vi "测试-掉线统计.vi"() -> ()   [LabVIEW 2017]
uses:
  <vilib>/Utility/miscctls.llb/LVRowAndColumnUnsignedTypeDef.ctl
panel:
  in  "标志-主动高亮":bool=TRUE
  in  "标志-刷新设备":bool=TRUE
  in  "清空记录":bool
  out "信号-高亮选中":bool=TRUE
  out "事件-新掉线记录":refnum<user-event>
  in  "掉线缓存":T1[](array[typedef])
  out "掉线记录":i32[](listbox)
  in  "设备":i32(listbox)
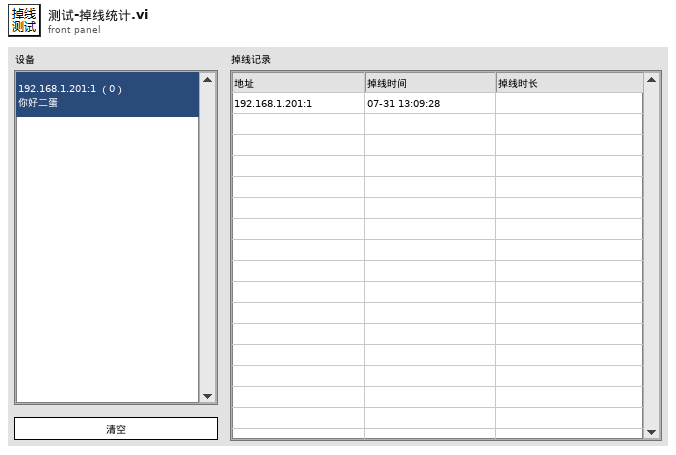
[diagram p1: front panel]
types:
  T1 = typedef "掉线缓存.ctl" = cluster{"掉线时长":string, "探头信息":cluster{"网络地址":string, "名称":string}, "掉线时间":timestamp, "记次":u16}
  T2 = typedef "LVRowAndColumnUnsignedTypeDef.ctl" = cluster{"Row":u32, "Column":u32}
  T3 = enum32{"Invalid", "Standard", "Closed", "Hidden", "Minimized", "Maximized"}
  T4 = typedef "探头属性.ctl" = cluster{"探头地址与信息":T5, "测量值":T8, "限值":T9, "探头状态":T10, "累积记录":T11, "报警方式":T12}
  T5 = typedef "探测器信息.ctl" = cluster{"网络地址":string, "名称":string, "备注":string, "累积剂量":dbl, "累积限值":dbl, "硬件剂量率限值":T6, "剂量率限值1":dbl, "剂量率限值2":dbl, "报警方式":T7}
  T6 = typedef "探头剂量率限值选择.ctl" = enum16{"一级限值", "二级限值"}
  T7 = typedef "报警方式选择.ctl" = enum16{"常报警", "自动静音", "手动静音"}
  T8 = typedef "测量值.ctl" = cluster{"时间":timestamp, "数值":dbl}
  T9 = typedef "剂量率限值.ctl" = cluster{"限值1":dbl, "限值2":dbl, "探头限值":T6}
  T10 = typedef "探头状态.ctl" = enum16{"正常", "离线", "禁用", "一级报警", "二级报警", "累积报警"}
  T11 = typedef "单条累积记录.ctl" = cluster{"起始时间":timestamp, "结束时间":timestamp, "累积剂量":dbl}
  T12 = typedef "报警方式.ctl" = cluster{"报警方式":T7, "延迟计时":u16, "报警中？":bool}
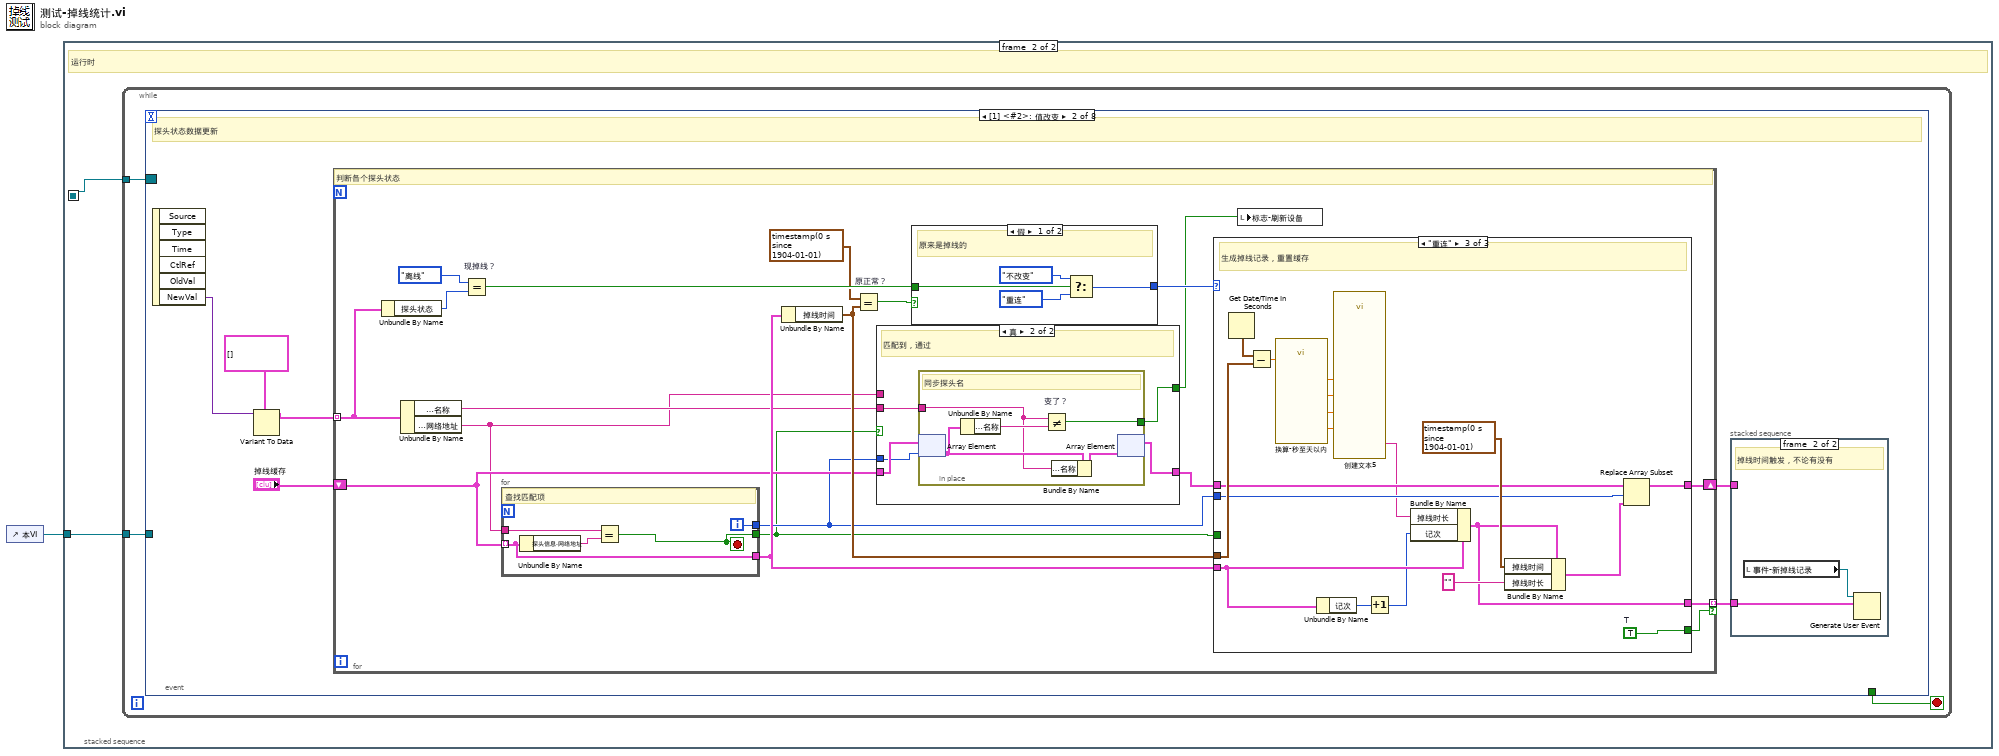
[diagram p0: block diagram]
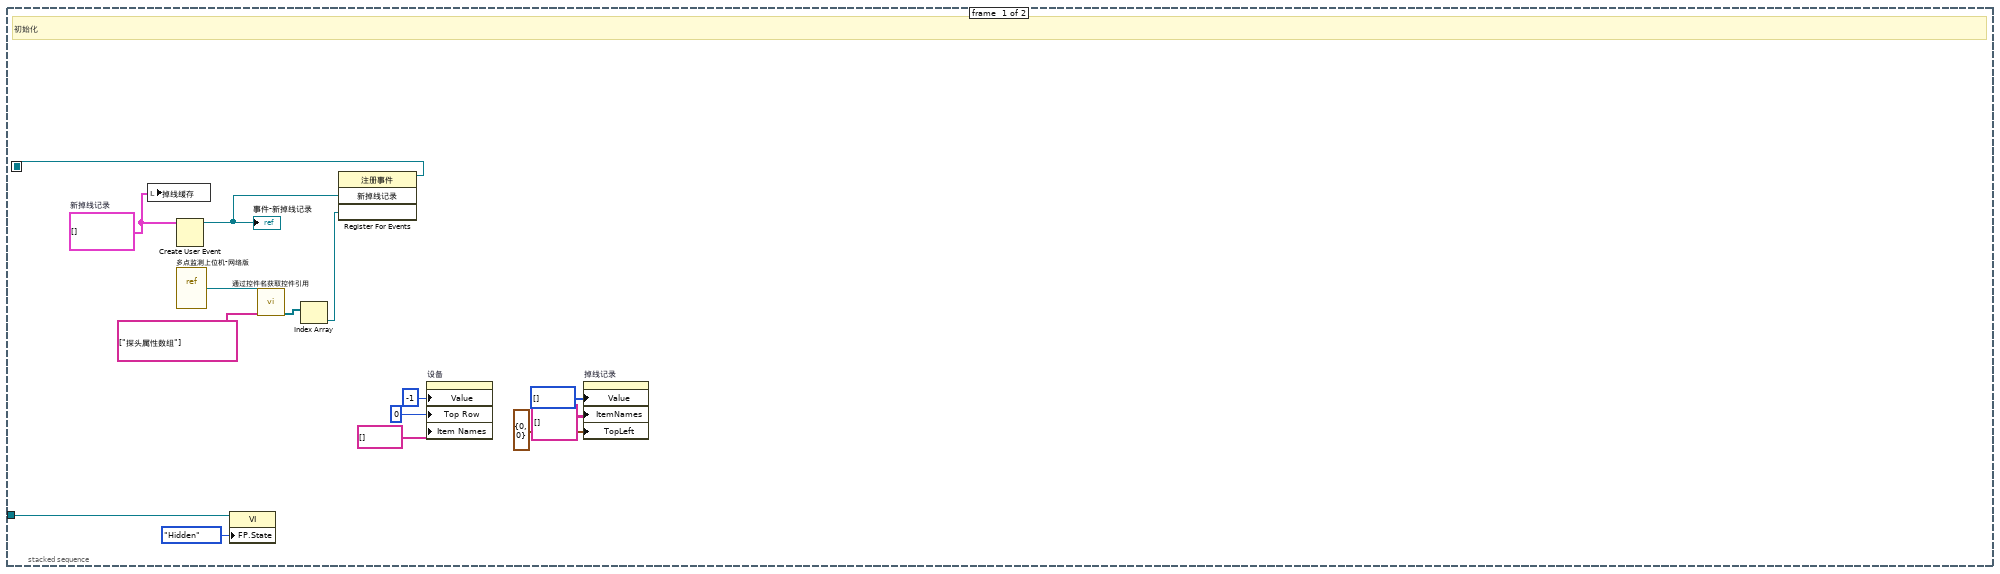
[diagram p2: hidden frame]
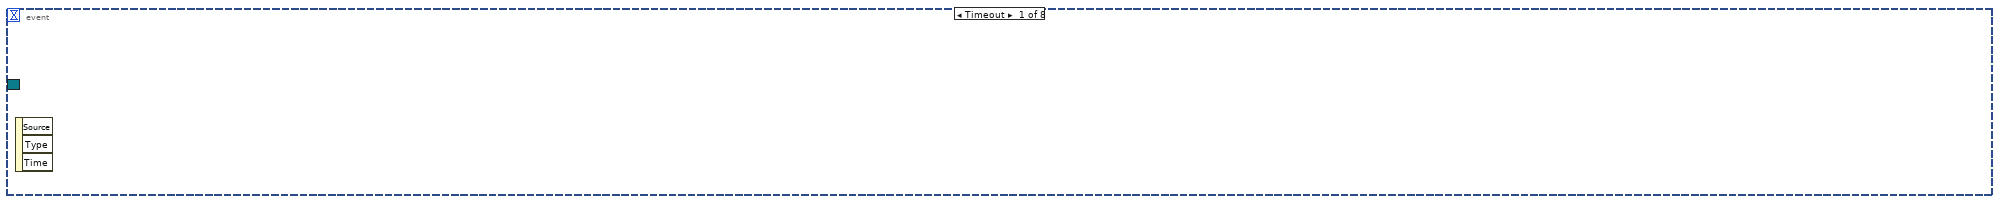
[diagram p3: hidden frame]
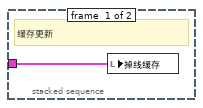
[diagram p4: hidden frame]
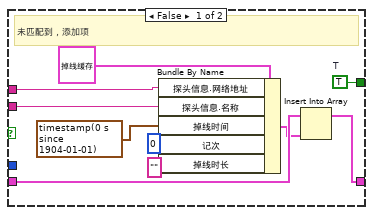
[diagram p5: hidden frame]
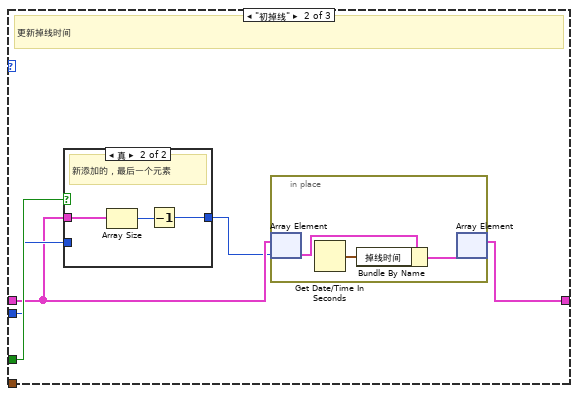
[diagram p7: hidden frame]
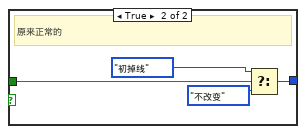
[diagram p9: hidden frame]
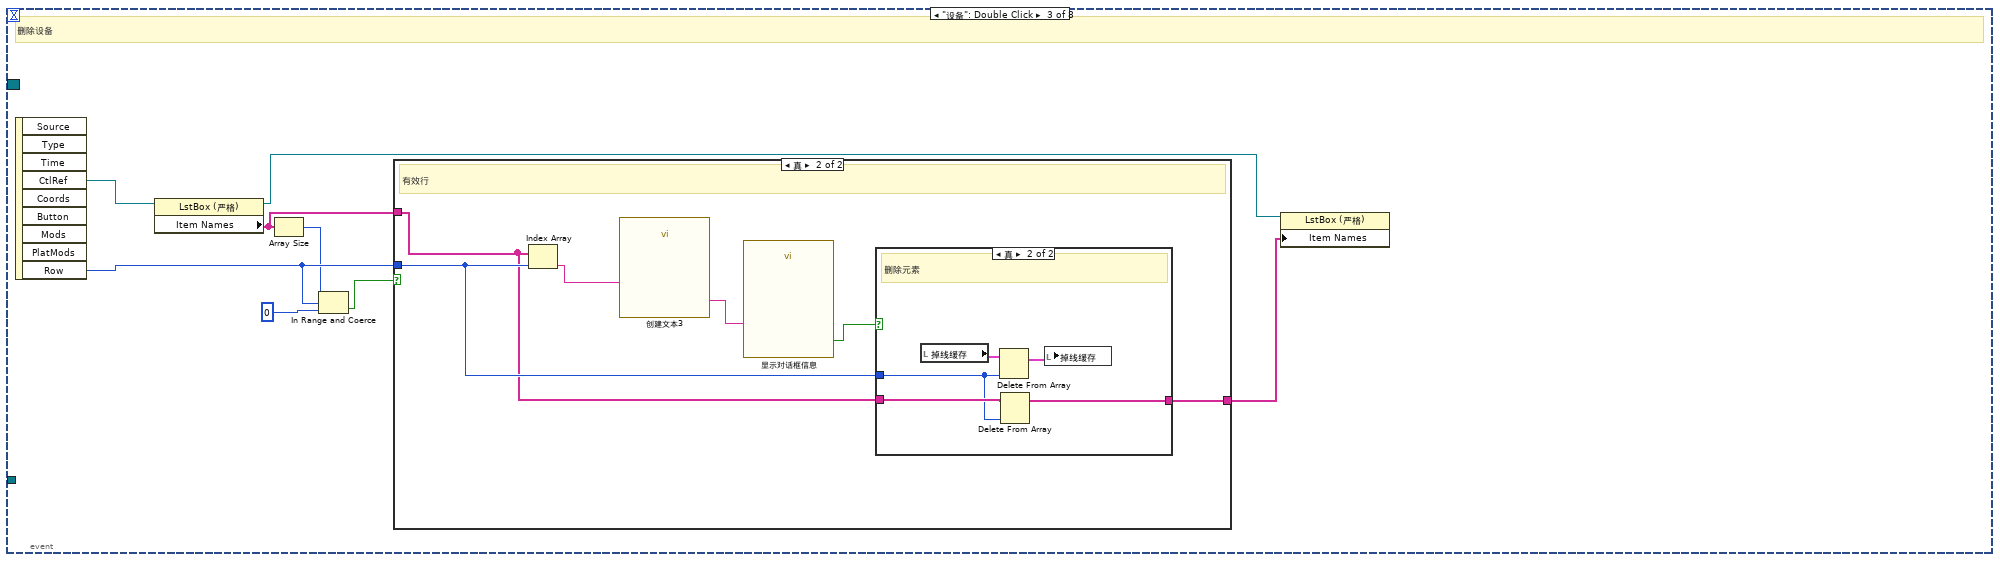
[diagram p10: hidden frame]
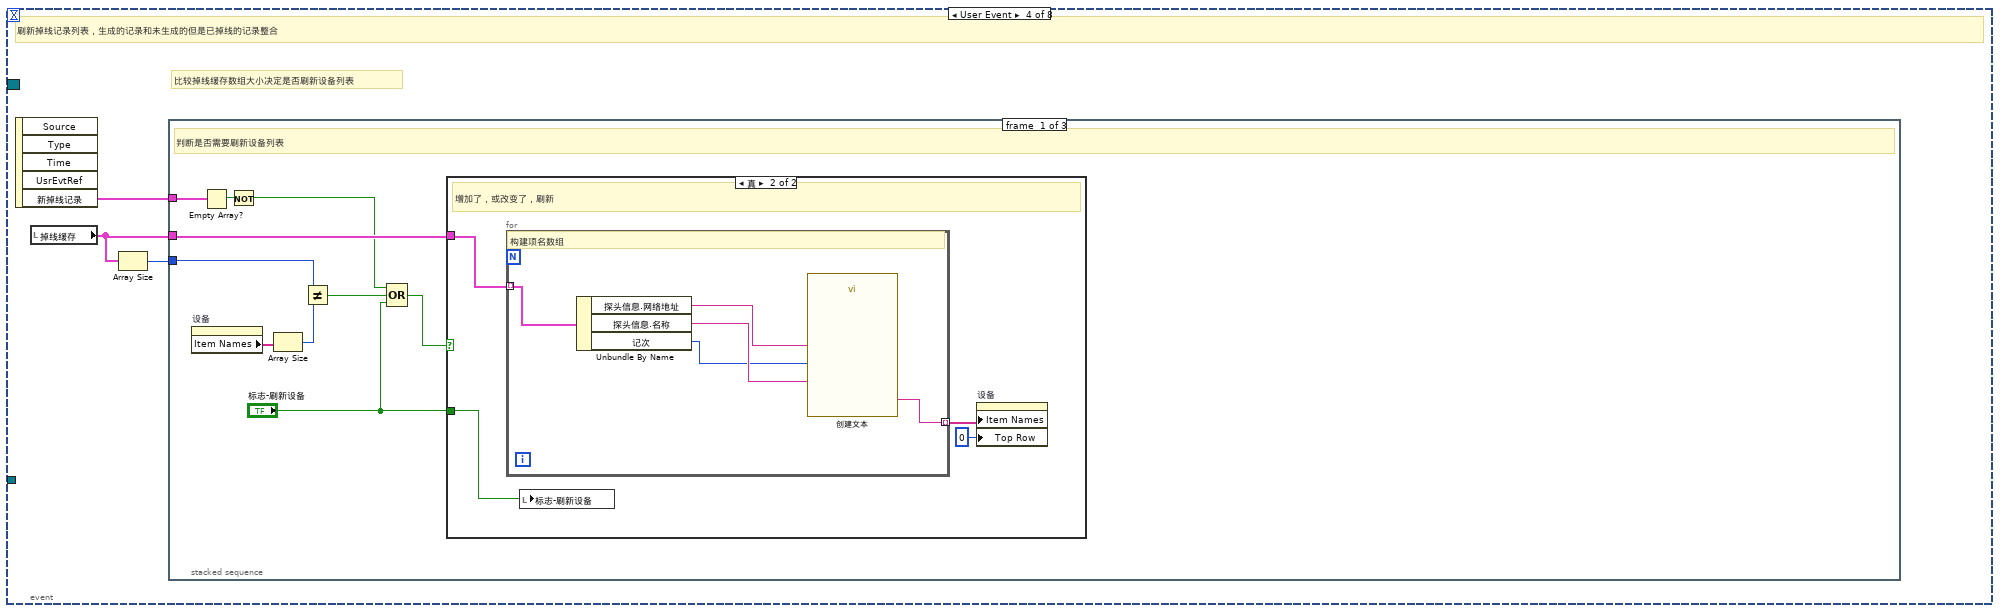
[diagram p13: hidden frame]
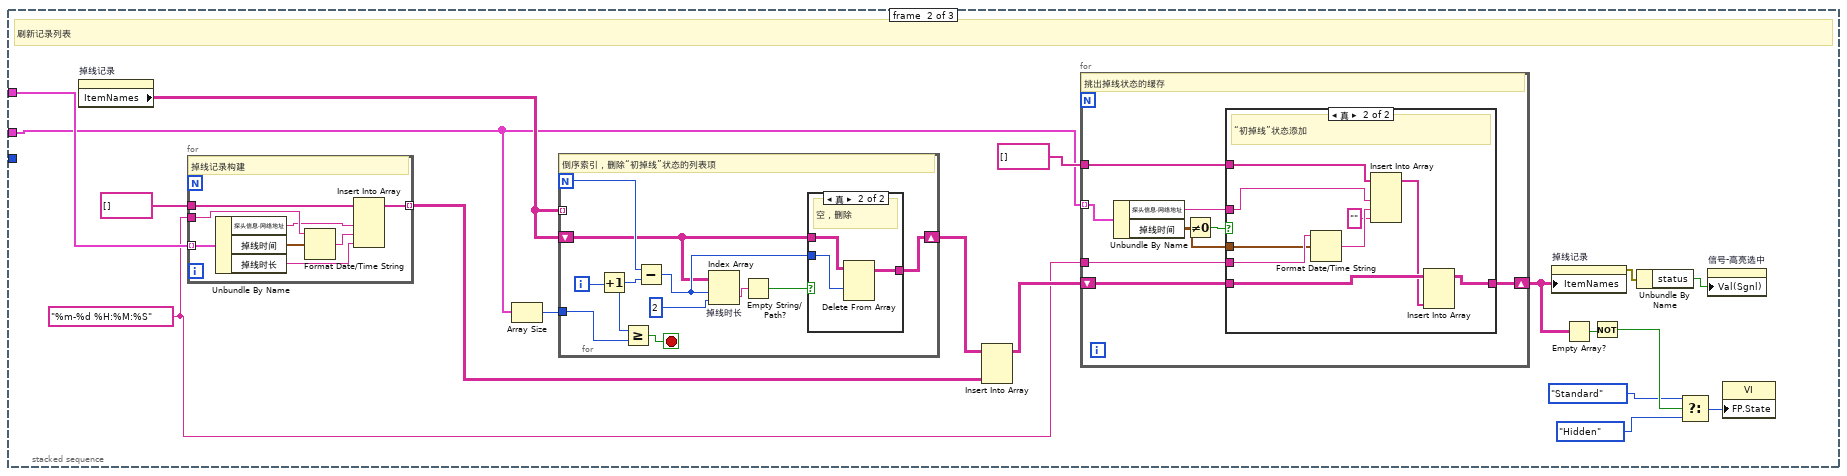
[diagram p15: hidden frame]
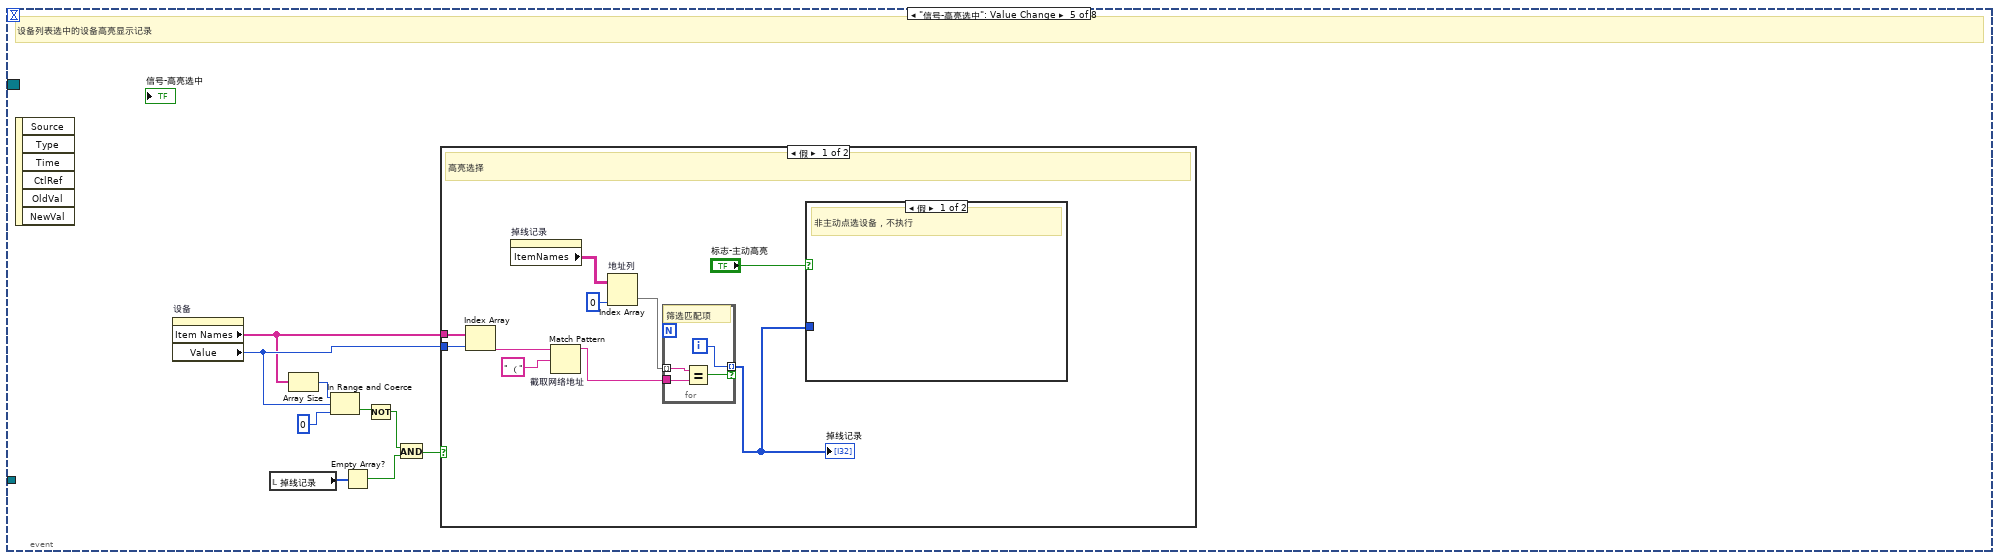
[diagram p19: hidden frame]
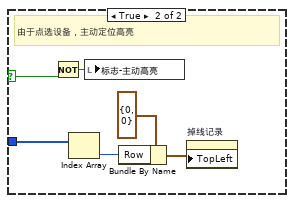
[diagram p20: hidden frame]
diagram:
  n1 = control-ref of="本VI"() -> (w1:refnum<vi>)
  n2 = stacked-sequence {
    seq-local: [w16 _] -> [_ w18]
    tunnel: w1 -> [w10 w17]
    frame #0 {
      w2 = T1[] []  # 新掉线记录
      # "初始化"
      n3 = local write "掉线缓存"(w2) -> ()
      n4 = Create User Event(user event datatype=w2) -> (user event=w3:refnum<user-event>)  [unwired: 1 in, 1 out]
      "事件-新掉线记录" <- w3
      n5 = vi-ref "多点监测上位机-网络版.vi"() -> (w15:refnum<vi>)
      n6 = property class="VI"(reference=w10, "FP.State"=T3."Hidden" ("前面板窗口:状态")) -> ()  [unwired: 1 in, 2 out]
      n7 = call "通过控件名获取控件引用.vi"("控件名数组"=string[] ["探头属性数组"], "VI引用"=w15) -> ("控件引用输出"=w13:refnum<vi>[])  [unwired: 7 in, 2 out]
      n8 = Index Array(array=w13) -> (element=w12:refnum<vi>)  [unwired: 1 in]
      n9 = register-events(w3, w12) -> (reference out=w16:refnum<event-registration>)  [unwired: 2 in, 1 out]
      n10 = property on="设备" class="LstBox (严格)"("Value"=-1 ("设备"), "Top Row"=0 ("顶行"), "Item Names"=string[] [] ("项名")) -> ()  [unwired: 2 in, 2 out]
      n11 = property on="掉线记录" class="MCListbox (严格)"("Value"=i32[] [] ("掉线记录"), "ItemNames"=string[][] [] ("项名"), "TopLeft"=T2 {"Row"=0, "Column"=0} ("左上可见单元格")) -> ()  [unwired: 2 in, 2 out]
    }
    frame #1 {
      # "运行时"
      n12 = while {
        tunnel: w18 -> [w21]
        tunnel: w17 -> [w19]
        stop <- w20 stop-if-true
        n13 = event shown="[1] <#2>: 值改变" {
          selector: w21 -> [_ _ _ _ _ _ _ _]
          dyn-events: _ -> [_ _ _ _ _ _ _ _]
          timeout: _ -> [_ _ _ _ _ _ _ _]
          tunnel: [_ _ _ _ _ _ _ w263] -> w20
          tunnel: w19 -> [_ _ _ _ _ w248 _ w262]
          event Timeout {
            n14 = event-data() -> ()  [unwired: 1 in, 3 out]
          }
          event Value Change {
            # "探头状态数据更新"
            n15 = event-data() -> ("NewVal"=w25:variant)  [unwired: 1 in, 5 out]
            n16 = Variant To Data(type=T4[] [] ("探头属性数组"), Variant=w25) -> (data=w23:T4[])  [unwired: 1 in, 1 out]
            n17 = for {
              tunnel: w23 -> [w48] mode=indexing
              shift-right: [w47] -> w26
              shift-left: "掉线缓存" -> [w36]
              tunnel: [w44] -> w27 mode=indexing if=w43
              # "判断各个探头状态"
              n18 = Unbundle By Name(w48) -> ("探头状态"=w49:T10)
              n19 = Unbundle By Name(w48) -> ("探头地址与信息.名称"=w37:string, "探头地址与信息.网络地址"=w32:string)
              n20 = Equal? "现掉线？"(x=探头状态."离线" ("探头状态"), y=w49) -> (x = y?=w45:bool)
              n21 = for {
                tunnel: w36 -> [w111] mode=indexing
                tunnel: w32 -> [w114]
                tunnel: [w110] -> w31
                tunnel: [w112] -> w34
                tunnel: [w111] -> w46
                i -> [w112]
                stop <- w110 stop-if-true
                # "查找匹配项"
                n22 = Unbundle By Name(w111) -> ("探头信息.网络地址"=w113:string)
                n23 = Equal?(x=w114, y=w113) -> (x = y?=w110:bool)
              }
              n24 = Unbundle By Name(w46) -> ("掉线时间"=w38:timestamp)
              n25 = Equal? "原正常？"(x=timestamp(0 s since 1904-01-01), y=w38) -> (x = y?=w40:bool)
              n26 = case shown="真" w31 {
                tunnel: w37 -> [w56 w62]
                tunnel: w36 -> [w55 w64]
                tunnel: [w54 w61] -> w35
                tunnel: w34 -> [_ w63]
                tunnel: [w52 w60] -> w33
                tunnel: w32 -> [w50 _]
                frame False {
                  w52 = TRUE  # T
                  # "未匹配到，添加项"
                  n27 = Bundle By Name(cluster=T1 {"掉线时长"="", "探头信息"={"网络地址"="", "名称"=""}, "掉线时间"=timestamp(0 s since 1904-01-01), "记次"=0} ("掉线记录 2"), "探头信息.网络地址"=w50, "探头信息.名称"=w56, "掉线时间"=timestamp(0 s since 1904-01-01), "记次"=u16 0, "掉线时长"="") -> (w53:T1)
                  n28 = Insert Into Array(array=w55, new element=w53) -> (w54:T1[])  [unwired: 1 in]
                }
                frame True {
                  # "匹配到，通过"
                  n29 = in-place {
                    in-place-border: w62 -> [w65]
                    in-place-border: [w66] -> w60
                    # "同步探头名"
                    n30 = in-place-array #1(w64, w63) -> (w68:T1)
                    n31 = Unbundle By Name(w68) -> ("探头信息.名称"=w67:string)
                    n32 = Not Equal? "变了？"(x=w65, y=w67) -> (x != y?=w66:bool)
                    n33 = Bundle By Name(cluster=w68, "探头信息.名称"=w65) -> (w69:T1)
                    n34 = in-place-array #1(w69) -> (w61:T1[])  [unwired: 1 out]
                  }
                }
              }
              n35 = case shown="假" w40 {
                tunnel: w45 -> [w105 w109]
                tunnel: [w102 w106] -> w39
                frame False {
                  # "原来是掉线的"
                  n36 = Select(t=enum16{"不改变", "初掉线", "重连"}."不改变", s=w105, f=enum16{"不改变", "初掉线", "重连"}."重连") -> (s? t:f=w102:enum16{"不改变", "初掉线", "重连"})
                }
                frame True {
                  # "原来正常的"
                  n37 = Select(t=enum16{"不改变", "初掉线", "重连"}."初掉线", s=w109, f=enum16{"不改变", "初掉线", "重连"}."不改变") -> (s? t:f=w106:enum16{"不改变", "初掉线", "重连"})
                }
              }
              n38 = case shown="\"重连\"" w39 {
                tunnel: [w70 w72 w91] -> w47
                tunnel: w35 -> [w70 w73 w94]
                tunnel: w34 -> [_ w74 w92]
                tunnel: w46 -> [_ _ w100]
                tunnel: w38 -> [_ _ w101]
                tunnel: [_ _ w90] -> w44
                tunnel: [_ _ w89] -> w43
                tunnel: w31 -> [_ w75 _]
                frame "不改变", Default {
                }
                frame "初掉线" {
                  # "更新掉线时间"
                  n39 = case shown="真" w75 {
                    tunnel: w73 -> [_ w81]
                    tunnel: w74 -> [w79 _]
                    tunnel: [w79 w80] -> w71
                    frame False {
                    }
                    frame True {
                      # "新添加的，最后一个元素"
                      n40 = Array Size(array=w81) -> (size(s)=w82:i32)
                      n41 = Decrement(x=w82) -> (x-1=w80:i32)
                    }
                  }
                  n42 = in-place {
                    n43 = in-place-array #2(w73, w71) -> (w77:T1)
                    n44 = Get Date/Time In Seconds() -> (seconds since 1Jan1904=w78:timestamp)
                    n45 = Bundle By Name(cluster=w77, "掉线时间"=w78) -> (w76:T1)
                    n46 = in-place-array #2(w76) -> (w72:T1[])  [unwired: 1 out]
                  }
                }
                frame "重连" {
                  w89 = TRUE  # T
                  # "生成掉线记录，重置缓存"
                  n47 = Get Date/Time In Seconds() -> (seconds since 1Jan1904=w99:timestamp)
                  n48 = Subtract(x=w99, y=w101) -> (x-y=w88:dbl)
                  n49 = call "换算-秒至天以内.vi"("秒"=w88) -> ("s"=w84:dbl, "m"=w85:dbl, "h"=w86:dbl, "d"=w87:dbl)  [unwired: 7 in]
                  n50 = Unbundle By Name(w100) -> ("记次"=w98:u16)
                  n51 = call "创建文本5"("秒"=w84, "天"=w87, "小时"=w86, "分"=w85) -> ("Result"=w83:string)  [unwired: 10 in, 1 out]
                  n52 = Increment(x=w98) -> (x+1=w97:u16)
                  n53 = Bundle By Name(cluster=w100, "掉线时长"=w83, "记次"=w97) -> (w90:T1)
                  n54 = Bundle By Name(cluster=w90, "掉线时间"=timestamp(0 s since 1904-01-01), "掉线时长"="") -> (w93:T1)
                  n55 = Replace Array Subset(array=w94, new element=w93, index=w92) -> (w91:T1[])
                }
              }
              n56 = local write "标志-刷新设备"(w33) -> ()
            }
            n57 = stacked-sequence {
              tunnel: w26 -> [w28 _]
              tunnel: w27 -> [_ w29]
              frame #0 {
                # "缓存更新"
                n58 = local write "掉线缓存"(w28) -> ()
              }
              frame #1 {
                # "掉线时间触发，不论有没有"
                n59 = local read "事件-新掉线记录"() -> (w30:refnum<user-event>)
                n60 = Generate User Event(user event=w30, event data cluster=w29) -> ()  [unwired: 2 in, 2 out]
              }
            }
          }
          event "设备": Double Click {
            # "删除设备"
            n61 = event-data() -> ("CtlRef"=w122:refnum<vi>, "Row"=w120:i32)  [unwired: 1 in, 7 out]
            n62 = property class="LstBox (严格)"(reference=w122) -> (reference out=w116:refnum<vi>, "Item Names"=w117:string[])  [unwired: 1 in, 1 out]
            n63 = Array Size(array=w117) -> (size(s)=w118:i32)
            n64 = In Range and Coerce(upper limit=w118, x=w120, lower limit=u16 0 ("下限")) -> (In Range?=w119:bool)  [unwired: 1 out]
            n65 = case shown="真" w119 {
              tunnel: w120 -> [_ w126]
              tunnel: w117 -> [w123 w125]
              tunnel: [w123 w124] -> w115
              frame False {
              }
              frame True {
                # "有效行"
                n66 = Index Array(array=w125, index=w126) -> (element=w129:string)
                n67 = call "创建文本3"("地址"=w129) -> ("Result"=w128:string)  [unwired: 13 in, 1 out]
                n68 = call "显示对话框信息"("Message"=w128) -> ("确定"=w127:bool)  [unwired: 9 in, 1 out]
                n69 = case shown="真" w127 {
                  tunnel: w126 -> [_ w132]
                  tunnel: w125 -> [w130 w133]
                  tunnel: [w130 w131] -> w124
                  frame False {
                  }
                  frame True {
                    # "删除元素"
                    n70 = local read "掉线缓存"() -> (w134:T1[])
                    n71 = Delete From Array(array=w134, index=w132) -> (array with subset deleted=w135:T1[])  [unwired: 1 in, 1 out]
                    n72 = Delete From Array(array=w133, index=w132) -> (array with subset deleted=w131:string[])  [unwired: 1 in, 1 out]
                    n73 = local write "掉线缓存"(w135) -> ()
                  }
                }
              }
            }
            n74 = property class="LstBox (严格)"(reference=w116, "Item Names"=w115) -> ()  [unwired: 1 in, 2 out]
          }
          event User Event {
            # "比较掉线缓存数组大小决定是否刷新设备列表"
            # "刷新掉线记录列表，生成的记录和未生成的但是已掉线的记录整合"
            n75 = event-data() -> ("新掉线记录"=w137:T1[])  [unwired: 1 in, 4 out]
            n76 = local read "掉线缓存"() -> (w136:T1[])
            n77 = Array Size(array=w136) -> (size(s)=w138:i32)
            n78 = stacked-sequence {
              tunnel: w138 -> [w146 _ _]
              tunnel: w136 -> [w144 w167 _]
              tunnel: w137 -> [w143 w175 _]
              frame #0 {
                # "判断是否需要刷新设备列表"
                n79 = property on="设备" class="LstBox (严格)"() -> ("Item Names"=w148:string[])  [unwired: 2 in, 2 out]
                n80 = Empty Array?(array=w143) -> (empty?=w142:bool)
                n81 = Not(x=w142) -> (.not. x?=w140:bool)
                n82 = Array Size(array=w148) -> (size(s)=w147:i32)
                n83 = Not Equal?(x=w146, y=w147) -> (x != y?=w145:bool)
                n84 = Compound Arithmetic op=OR(w140, w145, "标志-刷新设备") -> (w141:bool)
                n85 = case shown="真" w141 {
                  tunnel: w144 -> [_ w152]
                  tunnel: "标志-刷新设备" -> [_ w149]
                  frame False {
                    # "数量没变"
                  }
                  frame True {
                    # "增加了，或改变了，刷新"
                    n86 = for {
                      tunnel: w152 -> [w156] mode=indexing
                      tunnel: [w157] -> w151 mode=indexing
                      # "构建项名数组"
                      n87 = Unbundle By Name(w156) -> ("探头信息.网络地址"=w155:string, "探头信息.名称"=w154:string, "记次"=w153:u16)
                      n88 = call "创建文本"("网址"=w155, "记次"=w153, "名称"=w154) -> ("Result"=w157:string)  [unwired: 11 in, 1 out]
                    }
                    n89 = local write "标志-刷新设备"(w149) -> ()
                    n90 = property on="设备" class="LstBox (严格)"("Item Names"=w151, "Top Row"=0 ("顶行")) -> ()  [unwired: 2 in, 2 out]
                  }
                }
              }
              frame #1 {
                w170 = "%m-%d %H:%M:%S" ("时间格式字符串(%c)")
                # "刷新记录列表"
                n91 = property on="掉线记录" class="MCListbox (严格)"() -> ("ItemNames"=w168:string[][])  [unwired: 2 in, 2 out]
                n92 = for {
                  tunnel: w175 -> [w216] mode=indexing
                  tunnel: string[] [] ("添加的数组") -> [w215]
                  tunnel: w170 -> [w214]
                  tunnel: [w210] -> w173 mode=indexing
                  # "掉线记录构建"
                  n93 = Unbundle By Name(w216) -> ("探头信息.网络地址"=w209:string, "掉线时间"=w213:timestamp, "掉线时长"=w211:string)
                  n94 = Format Date/Time String(time format string (%c)=w214, seconds (now)=w213) -> (date/time string=w212:string)  [unwired: 1 in]
                  n95 = Insert Into Array(array=w215, new element #1=w209, new element #2=w212, new element #3=w211) -> (w210:string[])  [unwired: 1 in]
                }
                n96 = Array Size(array=w167) -> (size(s)=w166:i32)
                n97 = for {
                  N -> [w186]
                  shift-right: [w180] -> w172
                  shift-left: w168 -> [w181]
                  tunnel: w168 -> [_] mode=indexing
                  tunnel: w166 -> [w177]
                  i -> [w179]
                  stop <- w176 stop-if-true
                  # "倒序索引，删除“初掉线”状态的列表项"
                  n98 = Increment(x=w179) -> (x+1=w178:i32)
                  n99 = Greater Or Equal?(x=w178, y=w177) -> (x >= y?=w176:bool)
                  n100 = Subtract(x=w186, y=w178) -> (x-y=w182:i32)
                  n101 = Index Array "掉线时长"(array=w181, index (row)=w182, index (col)=2 ("索引")) -> (element=w184:string)
                  n102 = Empty String/Path?(string/path=w184) -> (empty?=w183:bool)
                  n103 = case shown="真" w183 {
                    tunnel: w182 -> [_ w190]
                    tunnel: w181 -> [w187 w189]
                    tunnel: [w187 w188] -> w180
                    frame False {
                    }
                    frame True {
                      # "空，删除"
                      n104 = Delete From Array(array=w189, index (row)=w190) -> (array with subset deleted=w188:string[][])  [unwired: 2 in, 1 out]
                    }
                  }
                }
                n105 = Insert Into Array(array=w172, new element=w173) -> (w171:string[][])  [unwired: 2 in]
                n106 = for {
                  tunnel: w167 -> [w196] mode=indexing
                  shift-right: [w191] -> w163
                  shift-left: w171 -> [w197]
                  tunnel: w170 -> [w194]
                  tunnel: string[] [] ("添加的数组") -> [w192]
                  # "挑出掉线状态的缓存"
                  n107 = Unbundle By Name(w196) -> ("探头信息.网络地址"=w195:string, "掉线时间"=w193:timestamp)
                  n108 = Not Equal To 0?(x=w193) -> (x != 0?=w198:bool)
                  n109 = case shown="真" w198 {
                    tunnel: w197 -> [w199 w208]
                    tunnel: w195 -> [_ w200]
                    tunnel: w194 -> [_ w207]
                    tunnel: w193 -> [_ w206]
                    tunnel: w192 -> [_ w205]
                    tunnel: [w199 w201] -> w191
                    frame False {
                      # "正常状态"
                    }
                    frame True {
                      # "“初掉线”状态添加"
                      n110 = Format Date/Time String(time format string (%c)=w207, seconds (now)=w206) -> (date/time string=w204:string)  [unwired: 1 in]
                      n111 = Insert Into Array(array=w205, new element #1=w200, new element #2=w204, new element #3="" ("新元素/子数组")) -> (w202:string[])  [unwired: 1 in]
                      n112 = Insert Into Array(array=w208, new element=w202) -> (w201:string[][])  [unwired: 2 in]
                    }
                  }
                }
                n113 = property on="掉线记录" class="MCListbox (严格)"("ItemNames"=w163) -> (error out=w165:errorcluster)  [unwired: 2 in, 1 out]
                n114 = Empty Array?(array=w163) -> (empty?=w162:bool)
                n115 = Not(x=w162) -> (.not. x?=w161:bool)
                n116 = Unbundle By Name(w165) -> ("status"=w164:bool)
                n117 = Select(t=T3."Standard" ("前面板窗口:状态"), s=w161, f=T3."Hidden" ("前面板窗口:状态")) -> (s? t:f=w158:T3)
                n118 = property on="信号-高亮选中" class="Bool (严格)"("Val(Sgnl)"=w164) -> ()  [unwired: 2 in, 2 out]
                n119 = property class="VI"("FP.State"=w158) -> ()  [unwired: 2 in, 2 out]
              }
              frame #2 {
              }
            }
          }
          event "信号-高亮选中": Value Change {
            # "设备列表选中的设备高亮显示记录"
            n120 = event-data() -> ()  [unwired: 1 in, 6 out]
            n121 = property on="设备" class="LstBox (严格)"() -> ("Item Names"=w223:string[], "Value"=w225:i32)  [unwired: 2 in, 2 out]
            n122 = local read "掉线记录"() -> (w221:i32[])
            n123 = Array Size(array=w223) -> (size(s)=w222:i32)
            n124 = In Range and Coerce(upper limit=w222, x=w225, lower limit=0 ("下限")) -> (In Range?=w219:bool)  [unwired: 1 out]
            n125 = Empty Array?(array=w221) -> (empty?=w220:bool)
            n126 = Not(x=w219) -> (.not. x?=w217:bool)
            n127 = And(x=w217, y=w220) -> (x .and. y?=w218:bool)
            n128 = case shown="假" w218 {
              tunnel: w225 -> [w228 _]
              tunnel: w223 -> [w227 _]
              frame False {
                # "高亮选择"
                n129 = Index Array(array=w227, index=w228) -> (element=w235:string)
                n130 = property on="掉线记录" class="MCListbox (严格)"() -> ("ItemNames"=w233:string[][])  [unwired: 2 in, 2 out]
                n131 = Match Pattern "截取网络地址"(string=w235, regular expression=" （" ("正则表达式")) -> (before substring=w230:string)  [unwired: 1 in, 3 out]
                n132 = Index Array "地址列"(array=w233, index (col)=0 ("禁用的索引 (列)")) -> (element=w231:string[])  [unwired: 1 in]
                n133 = for {
                  tunnel: w231 -> [w244] mode=indexing
                  tunnel: w230 -> [w245]
                  tunnel: [w243] -> w229 mode=indexing if=w242
                  i -> [w243]
                  # "筛选匹配项"
                  n134 = Equal?(x=w244, y=w245) -> (x = y?=w242:bool)
                }
                "掉线记录" <- w229
                n135 = case shown="假" "标志-主动高亮" {
                  selector: "标志-主动高亮" -> [_ w237]
                  tunnel: w229 -> [_ w241]
                  frame False {
                    # "非主动点选设备，不执行"
                  }
                  frame True {
                    # "由于点选设备，主动定位高亮"
                    n136 = Not(x=w237) -> (.not. x?=w236:bool)
                    n137 = Index Array(array=w241) -> (element=w238:i32)  [unwired: 1 in]
                    n138 = local write "标志-主动高亮"(w236) -> ()
                    n139 = Bundle By Name(cluster=T2 {"Row"=0, "Column"=0} ("左上可见单元格"), "Row"=w238) -> (w239:T2)
                    n140 = property on="掉线记录" class="MCListbox (严格)"("TopLeft"=w239) -> ()  [unwired: 2 in, 2 out]
                  }
                }
              }
              frame True {
                # "记录列表无高亮，且设备列表未选择设备，不执行"
              }
            }
          }
          event "清空记录": Value Change {
            n141 = event-data() -> ()  [unwired: 1 in, 6 out]
            n142 = property on="掉线记录" class="MCListbox (严格)"("ItemNames"=string[][] [] ("项名"), "TopLeft"=T2 {"Row"=0, "Column"=0} ("左上可见单元格"), "Value"=i32[] [] ("掉线记录")) -> (error out=w249:errorcluster)  [unwired: 2 in, 1 out]
            n143 = property class="VI"(reference=w248, error in=w249, "FP.State"=T3."Hidden" ("前面板窗口:状态")) -> ()  [unwired: 2 out]
            n144 = local read "掉线缓存"() -> (w247:T1[])
            n145 = for {
              tunnel: w247 -> [_] mode=indexing
              shift-right: [w254] -> w246
              shift-left: w247 -> [w256]
              i -> [w255]
              # "记次清零"
              n146 = in-place {
                n147 = in-place-array #3(w256, w255) -> (w259:T1)
                n148 = Bundle By Name(cluster=w259, "记次"=u16 0) -> (w258:T1)
                n149 = in-place-array #3(w258) -> (w254:T1[])  [unwired: 1 out]
              }
            }
            n150 = local write "掉线缓存"(w246) -> ()
          }
          event "设备": Value Change {
            w260 = TRUE  # T
            n151 = event-data() -> ()  [unwired: 1 in, 6 out]
            n152 = property on="信号-高亮选中" class="Bool (严格)"("Val(Sgnl)"=FALSE ("值(信号)")) -> ()  [unwired: 2 in, 2 out]
            n153 = local write "标志-主动高亮"(w260) -> ()
          }
          event Panel Close? {
            w263 = TRUE  # T
            n154 = event-data() -> ()  [unwired: 1 in, 4 out]
            n155 = disable-structure shown="禁用" {
              disable-tunnel: w262 -> [w264 _]
              frame Disabled {
                n156 = property class="VI"(reference=w264, "FP.State"=T3."Hidden" ("前面板窗口:状态")) -> ()  [unwired: 1 in, 2 out]
              }
              frame Enabled {
              }
            }
            n157 = event-data("Discard?"=w263) -> ()  [unwired: 1 in, 1 out]
          }
        }
      }
    }
  }
